vi "BuildMsg (Core).vi"(8 "error in (no error)":errorcluster, 10 "Msg to be build":string, 11 "CS++Actor in":refnum<class "CS++Actor.lvclass">) -> (0 "error out":errorcluster, 2 "ActiveMessageClass":refnum<vi>, 3 "CS++Actor out":refnum<class "CS++Actor.lvclass">)   [LabVIEW 2014, in "CS++Actor.lvlib" / "CS++Actor.lvclass"]
doc: "Core of the Build Msg command."
uses:
  CS++Actor.lvclass
  CS++Actor.lvclass/CS++Actor.ctl
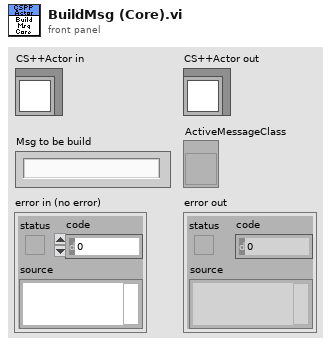
[diagram p1: front panel]
types:
  T1 = cluster{"Actor":cluster{"In":i32, "Out":i32}, "Error":cluster{"In":i32, "Out":i32}, "Terminals":cluster{"Position":enum16{"Left", "Top", "Bottom", "Right"}, "Terminal":i32}[]}
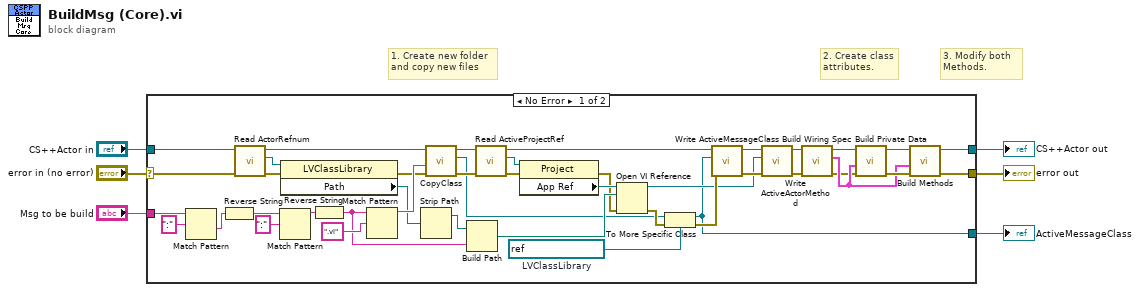
[diagram p0: block diagram]
diagram:
  # "3. Modify both\nMethods."
  # "2. Create class\nattributes."
  # "1. Create new folder\nand copy new files"
  n1 = case shown="No Error" "error in (no error)" {
    selector: "error in (no error)" -> [w27 w50]
    tunnel: [w21 w50] -> w5
    tunnel: [w22 w49] -> w3
    tunnel: "CS++Actor in" -> [w26 w49]
    tunnel: "Msg to be build" -> [w43 _]
    tunnel: [w7 _] -> w1
    frame No Error {
      w34 = refnum<vi> refnum  # LVClassLibrary
      n2 = Match Pattern(string=w43, regular expression=":") -> (after substring=w42:string)  [unwired: 1 in, 3 out]
      n3 = Reverse String(1:w42) -> (0:w48:string)
      n4 = call "Read ActorRefnum.vi"("error in (no error)"=w27, "CS++Actor in"=w26) -> ("error out"=w29:errorcluster, "ActorRefnum"=w28:refnum<vi>, "CS++Actor out"=w25:refnum<class "CS++Actor.lvclass">)  [unwired: 7 in]
      n5 = Match Pattern(string=w48, regular expression=":") -> (before substring=w46:string)  [unwired: 1 in, 3 out]
      n6 = property class="LVClassLibrary"(reference=w28, error in=w29) -> (error out=w24:errorcluster, "Path"=w23:path)  [unwired: 1 out]
      n7 = Reverse String(1:w46) -> (0:w41:string)
      n8 = Match Pattern(string=w41, regular expression=".vi") -> (before substring=w30:string)  [unwired: 1 in, 3 out]
      n9 = Strip Path(path=w23) -> (stripped path=w40:path)  [unwired: 1 out]
      n10 = call "CopyClass.vi"("error in (no error)"=w24, "Actor Method VI Name"=w30, "CS++Actor in"=w25) -> ("error out"=w32:errorcluster, "AddItemFromMemory"=w8:refnum<vi>, "CS++Actor out"=w31:refnum<class "CS++Actor.lvclass">)  [unwired: 5 in, 1 out]
      n11 = Build Path(base path=w40, name or relative path=w41) -> (appended path=w39:path)
      n12 = call "Read ActiveProjectRef.vi"("error in (no error)"=w32, "CS++Actor in"=w31) -> ("error out"=w36:errorcluster, "ActiveProjectRef"=w38:refnum<vi>, "CS++Actor out"=w18:refnum<class "CS++Actor.lvclass">)  [unwired: 7 in]
      n13 = property class="Project"(reference=w38, error in=w36) -> (error out=w35:errorcluster, "App Ref"=w37:refnum<vi>)  [unwired: 1 out]
      n14 = Open VI Reference(application reference (local)=w37, vi path=w39, error in (no error)=w35) -> (vi reference=w13:refnum<vi>, error out=w33:errorcluster)  [unwired: 3 in]
      n15 = To More Specific Class(target class=w34, reference=w8, error in=w33) -> (specific class reference=w7:refnum<vi>, error out=w17:errorcluster)
      n16 = call "Write ActiveMessageClass.vi"("error in (no error)"=w17, "ActiveMessageClass"=w7, "CS++Actor in"=w18) -> ("error out"=w16:errorcluster, "CS++Actor out"=w15:refnum<class "CS++Actor.lvclass">)  [unwired: 7 in]
      n17 = call "Write ActiveActorMethod.vi"("error in (no error)"=w16, "ActiveActorMethod"=w13, "CS++Actor in"=w15) -> ("error out"=w14:errorcluster, "CS++Actor out"=w12:refnum<class "CS++Actor.lvclass">)  [unwired: 7 in]
      n18 = call "Build Wiring Spec.vi"("error in (no error)"=w14, "CS++Actor in"=w12) -> ("error out"=w10:errorcluster, "Wiring Spec"=w19:T1, "CS++Actor out"=w9:refnum<class "CS++Actor.lvclass">)  [unwired: 7 in]
      n19 = call "Build Private Data.vi"("error in (no error)"=w10, "Wiring Spec"=w19, "CS++Actor in"=w9) -> ("error out"=w20:errorcluster, "CS++Actor out"=w11:refnum<class "CS++Actor.lvclass">)  [unwired: 7 in]
      n20 = call "Build Methods.vi"("error in (no error)"=w20, "Wiring Spec"=w19, "CS++Actor in"=w11) -> ("error out"=w21:errorcluster, "CS++Actor out"=w22:refnum<class "CS++Actor.lvclass">)  [unwired: 7 in]
    }
    frame Error {
    }
  }
  "error out" <- w5
  "CS++Actor out" <- w3
  "ActiveMessageClass" <- w1
